vi "HHMI - Delay if in simulation mode.vi"(10 "Count(mSec)":u32=10) -> ()   [LabVIEW 2013]
doc: "Wait a number of milliseconds only if being run on the Development Computer. This prevents loops taking all the CPU resources."
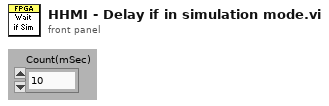
[diagram p1: front panel]
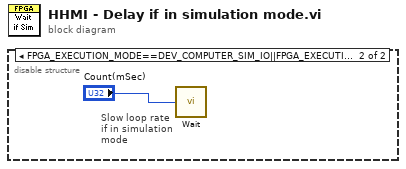
[diagram p0: block diagram]
diagram:
  n1 = disable-structure shown="FPGA_EXECUTION_MODE==DEV_COMPUTER_SIM_IO||FPGA_EXECUTION_MODE==DEV_COMPUTER_REAL_IO" {
    frame condition #0 {
    }
    frame condition #1 (active) {
      # "Slow loop rate\nif in simulation\nmode"
      n2 = call "Wait"("Count(mSec)"="Count(mSec)") -> ()  [unwired: 1 out]
    }
  }
